vi "UDP Multicast Receiver.vi"(3 "error in (no error)":errorcluster, 5 "UDP Network Connection Refnum":refnum<k16>) -> (0 "error out":errorcluster, 2 "Data Received":string)   [LabVIEW 2011]
doc: "UDP multicast will allow LabVIEW to send data to a multicast group or to receive data sent to a multicast group. In LabVIEW, UDP multicast is used in very much the same way as UDP. The main difference is there are two new parameters, TTL and Multicast Address, on the UDP Multicast Open. \n\nWhen sending to a multicast group the default time-to-live (TTL) is 1, which only allows the packet to go to the local subnet. When a router receives a multicast packet, it decrements the packets TTL, and if the TTL is greater than 0, forwards the packet to other routers.\nA multicast group is defined by having a multicast IP address in the range 224.0.0.0-239.255.255.255."
panel:
  in  "stop":bool
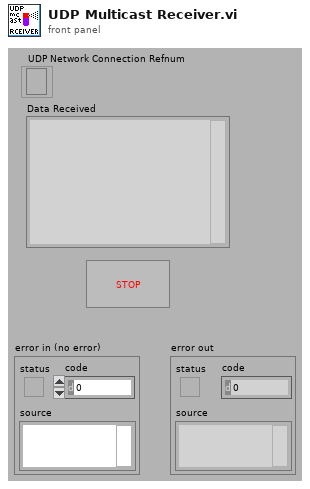
[diagram p1: front panel]
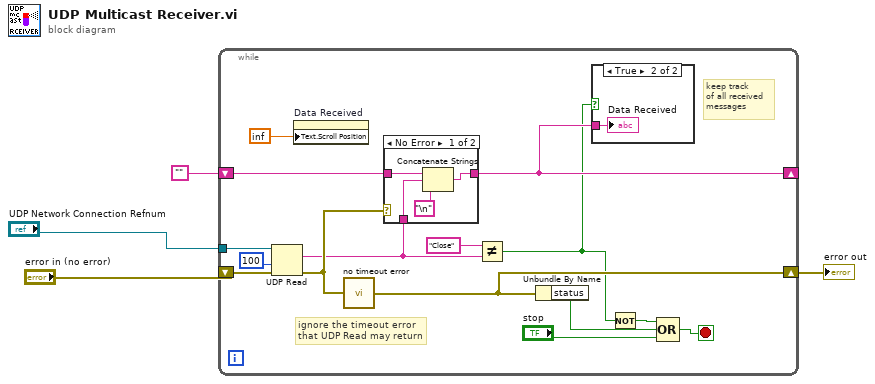
[diagram p0: block diagram]
diagram:
  n1 = while {
    tunnel: "UDP Network Connection Refnum" -> [w19]
    shift-right: [w9] -> _
    shift-left: "" -> [w18]
    shift-right: [w11] -> w3
    shift-left: "error in (no error)" -> [w13]
    stop <- w15 stop-if-true
    # "ignore the timeout error\nthat UDP Read may return"
    # "keep track\nof all received\nmessages"
    n2 = UDP Read(connection ID=w19, timeout ms (25000)=100, 8:w13) -> (data out=w6:string, error out=w10:errorcluster)  [unwired: 4 out]
    n3 = property on="Data Received" class="Str"("Text.Scroll Position"=inf) -> ()  [unwired: 2 in, 2 out]
    n4 = call "no timeout error.vi"("error in (no error)"=w10) -> ("error out"=w11:errorcluster)
    n5 = case shown="No Error" w10 {
      tunnel: w18 -> [w24 w25]
      tunnel: w6 -> [w23 _]
      tunnel: [w21 w25] -> w9
      frame No Error {
        n6 = Concatenate Strings(w24, w23, "\n") -> (w21:string)
      }
      frame Error {
      }
    }
    n7 = Not Equal?(x="Close", y=w6) -> (x != y?=w5:bool)
    n8 = Unbundle By Name(w11) -> ("status"=w17:bool)
    n9 = case shown="True" w5 {
      tunnel: w9 -> [_ w20]
      frame False {
      }
      frame True {
        "Data Received" <- w20
      }
    }
    n10 = Not(x=w5) -> (.not. x?=w8:bool)
    n11 = Compound Arithmetic op=OR(w8, w17, "stop") -> (w15:bool)
  }
  "error out" <- w3
